vi "GV line clock gate.vi"() -> ()   [LabVIEW 2017]
panel:
  out "Line clock gate":bool
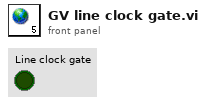
[diagram p1: front panel]
diagram:
